vi "terminate.vi"(8 "error in (no error)":errorcluster, 11 "GenericPlugin in":refnum<class "ClockDL100201DAQmx.lvclass">) -> (0 "error out":errorcluster, 3 "GenericPlugin out":refnum<class "ClockDL100201DAQmx.lvclass">)   [LabVIEW 2010, in "ClockDL100201DAQmx.lvclass"]
doc: "The dynamic dispatch version of this VI terminates the plug-in object by releasing all of its resources."
uses:
  ClockDL100201DAQmx.lvclass
  ClockDL100201DAQmx.lvclass/ClockDL100201DAQmx.ctl
  GenericClock/GenericClock/GenericClock.lvclass
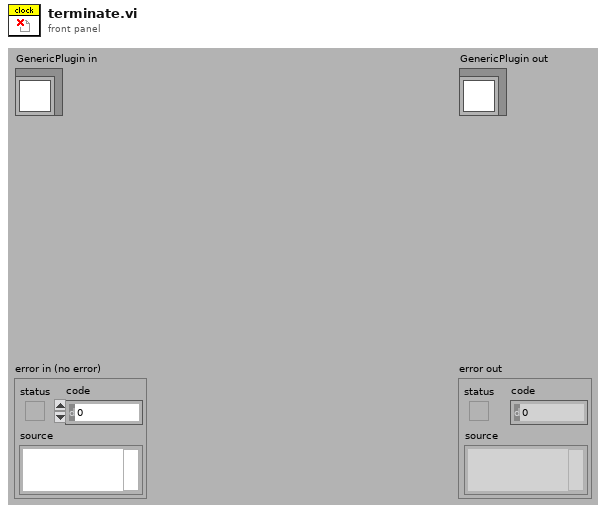
[diagram p1: front panel]
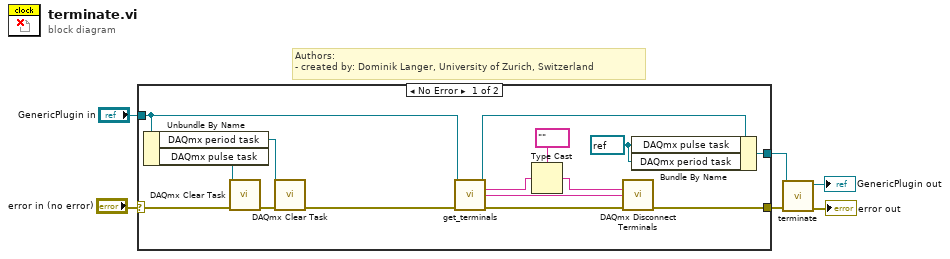
[diagram p0: block diagram]
diagram:
  # "Authors: \n- created by: Dominik Langer, University of Zurich, Switzerland"
  n1 = case shown="No Error" "error in (no error)" {
    selector: "error in (no error)" -> [w20 w22]
    tunnel: [w15 w22] -> w3
    tunnel: "GenericPlugin in" -> [w18 w23]
    tunnel: [w19 w23] -> w1
    frame No Error {
      w7 = refnum<k21> refnum ("DAQmx task")
      n2 = Unbundle By Name(w18) -> ("DAQmx period task"=w8:refnum<k21>, "DAQmx pulse task"=w21:refnum<k21>)
      n3 = call <vilib>:"DAQmx Clear Task.vi"("task in"=w21, "error in"=w20) -> ("error out"=w10:errorcluster)  [unwired: 13 in]
      n4 = call <vilib>:"DAQmx Clear Task.vi"("task in"=w8, "error in"=w10) -> ("error out"=w9:errorcluster)  [unwired: 13 in]
      n5 = call-dynamic "get_terminals.vi"("ClockDL100201DAQmx in"=w18, "error in (no error)"=w9) -> ("ClockDL100201DAQmx out"=w17:refnum<class "ClockDL100201DAQmx.lvclass">, "pulse counter"=w12:tag, "trigger source"=w14:tag, "error out"=w16:errorcluster)  [unwired: 9 in, 1 out]
      n6 = Type Cast(type=tag "" ("source terminal"), x=w12) -> (*(type *) &x=w11:tag)
      n7 = call <vilib>:"DAQmx Disconnect Terminals.vi"("source terminal"=w11, "destination terminal"=w14, "error in"=w16) -> ("error out"=w15:errorcluster)  [unwired: 12 in]
      n8 = Bundle By Name(cluster=w17, "DAQmx pulse task"=w7, "DAQmx period task"=w7) -> (w19:refnum<class "ClockDL100201DAQmx.lvclass">)
    }
    frame Error {
    }
  }
  n9 = call-parent "terminate.vi"("error in (no error)"=w3, "GenericPlugin in"=w1) -> ("error out"=→"error out":errorcluster, "GenericPlugin out"=→"GenericPlugin out":refnum<class "ClockDL100201DAQmx.lvclass">)  [unwired: 8 in]
